vi "johnson counter.vi"() -> ()   [LabVIEW 2020]
panel:
  in  "CLOCK":bool
  out "QC":bool
  out "QB":bool
  out "QA":bool
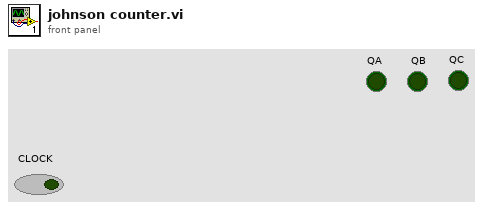
[diagram p1: front panel]
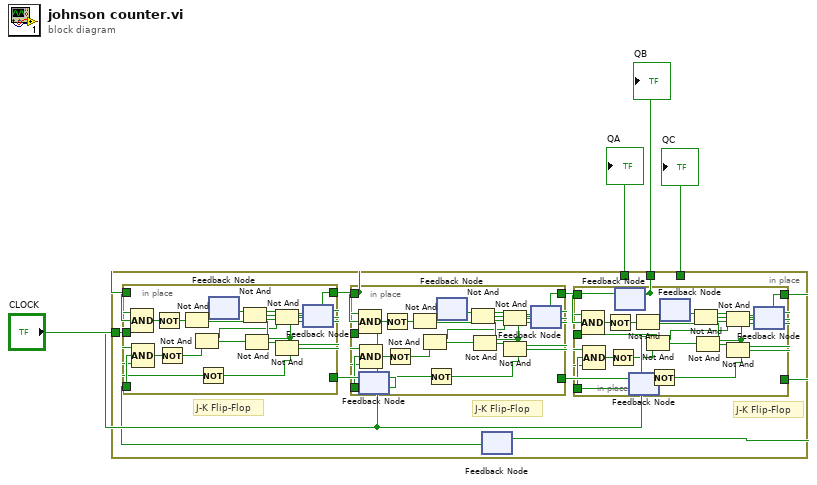
[diagram p0: block diagram]
diagram:
  n1 = in-place {
    in-place-border: "CLOCK" -> [w15]
    in-place-border: [w14] -> w3
    in-place-border: [w11] -> w2
    in-place-border: [w5] -> w1
    # "J-K Flip-Flop"
    # "J-K Flip-Flop"
    # "J-K Flip-Flop"
    n2 = feedback #1() -> (w9:bool)  [unwired: 1 in]
    n3 = feedback #2() -> (w12:bool)  [unwired: 1 in]
    n4 = feedback #3() -> (w5:bool)  [unwired: 1 in]
    n5 = feedback #4() -> (w7:bool)  [unwired: 1 in]
    n6 = in-place {
      in-place-border: w5 -> [w26]
      in-place-border: w7 -> [w25]
      in-place-border: w15 -> [w23]
      in-place-border: [w21] -> w13
      in-place-border: [w20] -> w11
      n7 = Not(x=w23) -> (.not. x?=w24:bool)
      n8 = feedback #5() -> (w29:bool)  [unwired: 1 in]
      n9 = Not And(1:w24, 2:w29) -> (0:w28:bool)
      n10 = feedback #6() -> (w20:bool)  [unwired: 1 in]
      n11 = Compound Arithmetic op=AND(w23, w25, w20) -> (w17:bool)
      n12 = Not(x=w17) -> (.not. x?=w16:bool)
      n13 = Not And(1:w16, 2:w29) -> (0:w31:bool)
      n14 = Not And(1:w31, 2:w24) -> (0:w27:bool)
      n15 = Not And(1:w27, 2:w20) -> (0:w21:bool)
      n16 = Compound Arithmetic op=AND(w21, w26, w23) -> (w19:bool)
      n17 = Not(x=w19) -> (.not. x?=w18:bool)
      n18 = Not And(1:w31, 2:w18) -> (0:w30:bool)
      n19 = feedback-in #5(w30) -> ()
      n20 = Not And(1:w21, 2:w28) -> (0:w22:bool)
      n21 = feedback-in #6(w22) -> ()
    }
    n22 = in-place {
      in-place-border: w13 -> [w58]
      in-place-border: w12 -> [w57]
      in-place-border: w15 -> [w55]
      in-place-border: [w53] -> w10
      in-place-border: [w52] -> w14
      n23 = Not(x=w55) -> (.not. x?=w56:bool)
      n24 = feedback #7() -> (w61:bool)  [unwired: 1 in]
      n25 = Not And(1:w56, 2:w61) -> (0:w60:bool)
      n26 = feedback #8() -> (w52:bool)  [unwired: 1 in]
      n27 = Compound Arithmetic op=AND(w55, w57, w52) -> (w49:bool)
      n28 = Not(x=w49) -> (.not. x?=w48:bool)
      n29 = Not And(1:w48, 2:w61) -> (0:w63:bool)
      n30 = Not And(1:w63, 2:w56) -> (0:w59:bool)
      n31 = Not And(1:w59, 2:w52) -> (0:w53:bool)
      n32 = Compound Arithmetic op=AND(w53, w58, w55) -> (w51:bool)
      n33 = Not(x=w51) -> (.not. x?=w50:bool)
      n34 = Not And(1:w63, 2:w50) -> (0:w62:bool)
      n35 = feedback-in #7(w62) -> ()
      n36 = Not And(1:w53, 2:w60) -> (0:w54:bool)
      n37 = feedback-in #8(w54) -> ()
    }
    n38 = in-place {
      in-place-border: w14 -> [w42]
      in-place-border: w9 -> [w41]
      in-place-border: w15 -> [w39]
      in-place-border: [w37] -> w8
      in-place-border: [w36] -> w6
      n39 = Not(x=w39) -> (.not. x?=w40:bool)
      n40 = feedback #9() -> (w45:bool)  [unwired: 1 in]
      n41 = Not And(1:w40, 2:w45) -> (0:w44:bool)
      n42 = feedback #10() -> (w36:bool)  [unwired: 1 in]
      n43 = Compound Arithmetic op=AND(w39, w41, w36) -> (w33:bool)
      n44 = Not(x=w33) -> (.not. x?=w32:bool)
      n45 = Not And(1:w32, 2:w45) -> (0:w47:bool)
      n46 = Not And(1:w47, 2:w40) -> (0:w43:bool)
      n47 = Not And(1:w43, 2:w36) -> (0:w37:bool)
      n48 = Compound Arithmetic op=AND(w37, w42, w39) -> (w35:bool)
      n49 = Not(x=w35) -> (.not. x?=w34:bool)
      n50 = Not And(1:w47, 2:w34) -> (0:w46:bool)
      n51 = feedback-in #9(w46) -> ()
      n52 = Not And(1:w37, 2:w44) -> (0:w38:bool)
      n53 = feedback-in #10(w38) -> ()
    }
    n54 = feedback-in #1(w10) -> ()
    n55 = feedback-in #2(w11) -> ()
    n56 = feedback-in #3(w6) -> ()
    n57 = feedback-in #4(w8) -> ()
  }
  "QA" <- w3
  "QB" <- w1
  "QC" <- w2
